vi "DetectCollisionSmoother.vi"(0 "Goal":dbl[](array[numeric]), 4 "Initial State":dbl[](array[numeric]), 6 "enemy_robots":T1[](array[typedef]), 7 "Robot in":T1={"id"=0, "function"=enum."Attacker", "x"=0.0, "y"=0.0, "orientation"=0.0, "v_tangent"=0.0, "v_normal"=0.0, "v_ang"=0.0, "kick_x"=0.0, "kick_z"=0.0, "dribble"=FALSE, "Timestamp"=timestamp(0 s since 1904-01-01), "estimatives"={"est_v_tangent"=0.0, "est_v_normal"=0.0, "est_vx"=0.0, "est_vy"=0.0, "Pos Robot Est"=[]}, "dest_x_kick"=0.0, "dest_y_kick"=0.0, "Gap Coord"=[], "States"=enum."Pass", "Path "=[], "Path  Smooth"=[], "Dest"=[], "vx_desired"=0.0, "vy_desired"=0.0, "slowBehavior"=FALSE, "VSSStates"=enum."Pass"}, 8 "SegmentPointB":dbl[](array[numeric]), 9 "SegmentPointA":dbl[](array[numeric]), 10 "ball":dbl[](array[numeric]), 11 "ignoreBall?":bool) -> (3 "Is there colision?":bool)   [LabVIEW 2023]
uses:
  Vision_class/Old vision/Controls/AI Robot.ctl
  Vision_class/Old vision/Controls/Functions Enum.ctl
  Vision_class/Old vision/Controls/AttackerStates.ctl
  Vision_class/Old vision/Controls/PathDests.ctl
  Vision_class/Old vision/Controls/PathDest.ctl
  Navigation/VSSNavigation/VSSAttackerStates.ctl
panel:
  in  "our_robots":T1[](array[typedef])
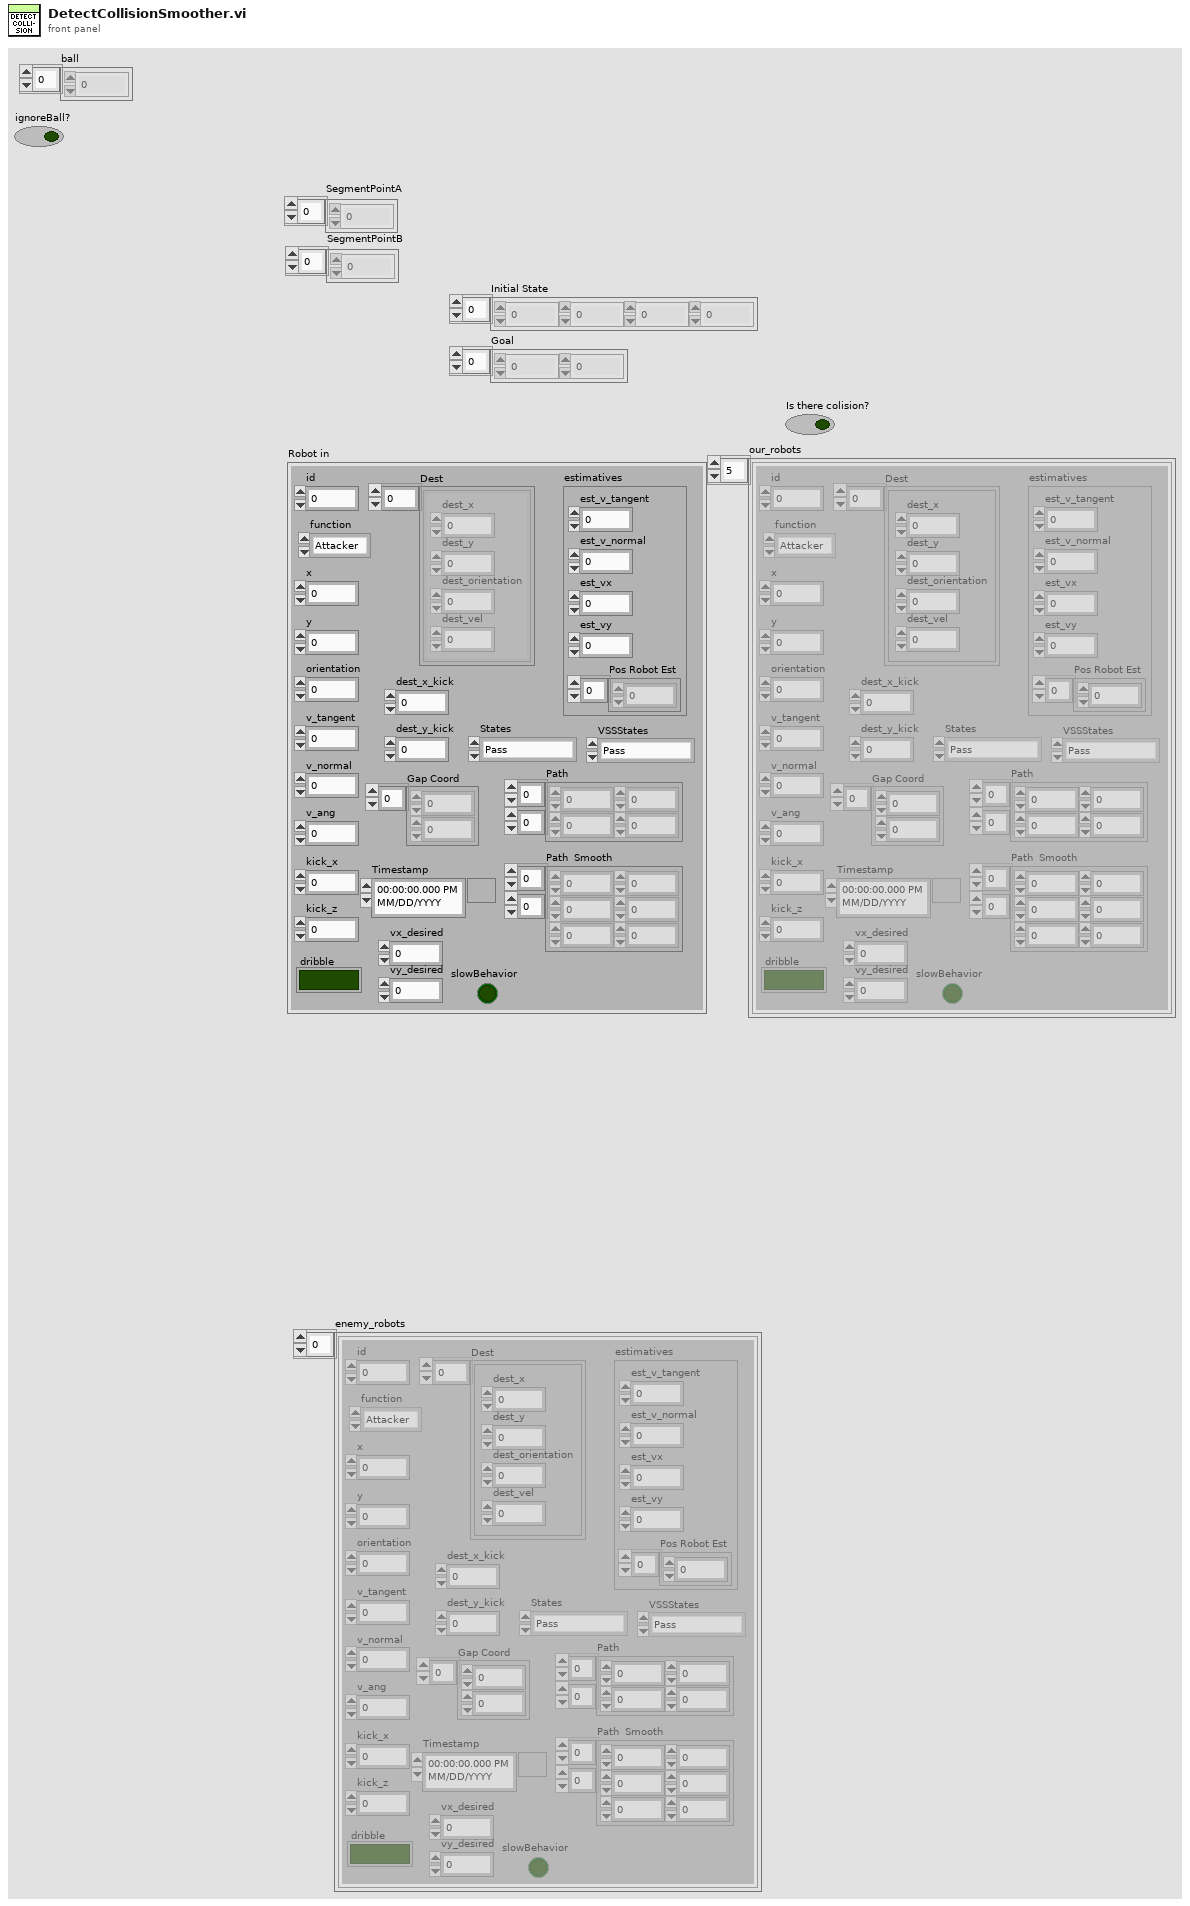
[diagram p1: front panel]
types:
  T1 = typedef "AI Robot.ctl" = cluster{"id":u32, "function":T2, "x":dbl, "y":dbl, "orientation":dbl, "v_tangent":dbl, "v_normal":dbl, "v_ang":dbl, "kick_x":dbl, "kick_z":dbl, "dribble":bool, "Timestamp":timestamp, "estimatives":cluster{"est_v_tangent":dbl, "est_v_normal":dbl, "est_vx":dbl, "est_vy":dbl, "Pos Robot Est":dbl[]}, "dest_x_kick":dbl, "dest_y_kick":dbl, "Gap Coord":dbl[], "States":T3, "Path ":dbl[][], "Path  Smooth":dbl[][], "Dest":T4, "vx_desired":dbl, "vy_desired":dbl, "slowBehavior":bool, "VSSStates":T6}
  T2 = typedef "Functions Enum.ctl" = enum16{"2nd Striker", "Attacker", "Goalie", "Defender", "Striker", "Goto 0", "Dummy", "Kicker", "ZigZag 0", "ZigZag 1", "ZigZag 2", "ZigZag 3", "ZigZag 4", "ZigZag 5", "ZigZag 6", "ZigZag 7", "ZigZag 8", ""}
  T3 = typedef "AttackerStates.ctl" = enum16{"Pass", "GoToTangent", "BallGetting", "GoToKick", ""}
  T4 = typedef "PathDests.ctl" = T5[]
  T5 = typedef "PathDest.ctl" = cluster{"dest_x":dbl, "dest_y":dbl, "dest_orientation":dbl, "dest_vel":dbl}
  T6 = typedef "VSSAttackerStates.ctl" = enum16{"Pass", "GoToTangent", "BallGetting", "GoToKick", "Rotate anti-clockwise", "Rotate Clockwise", ""}
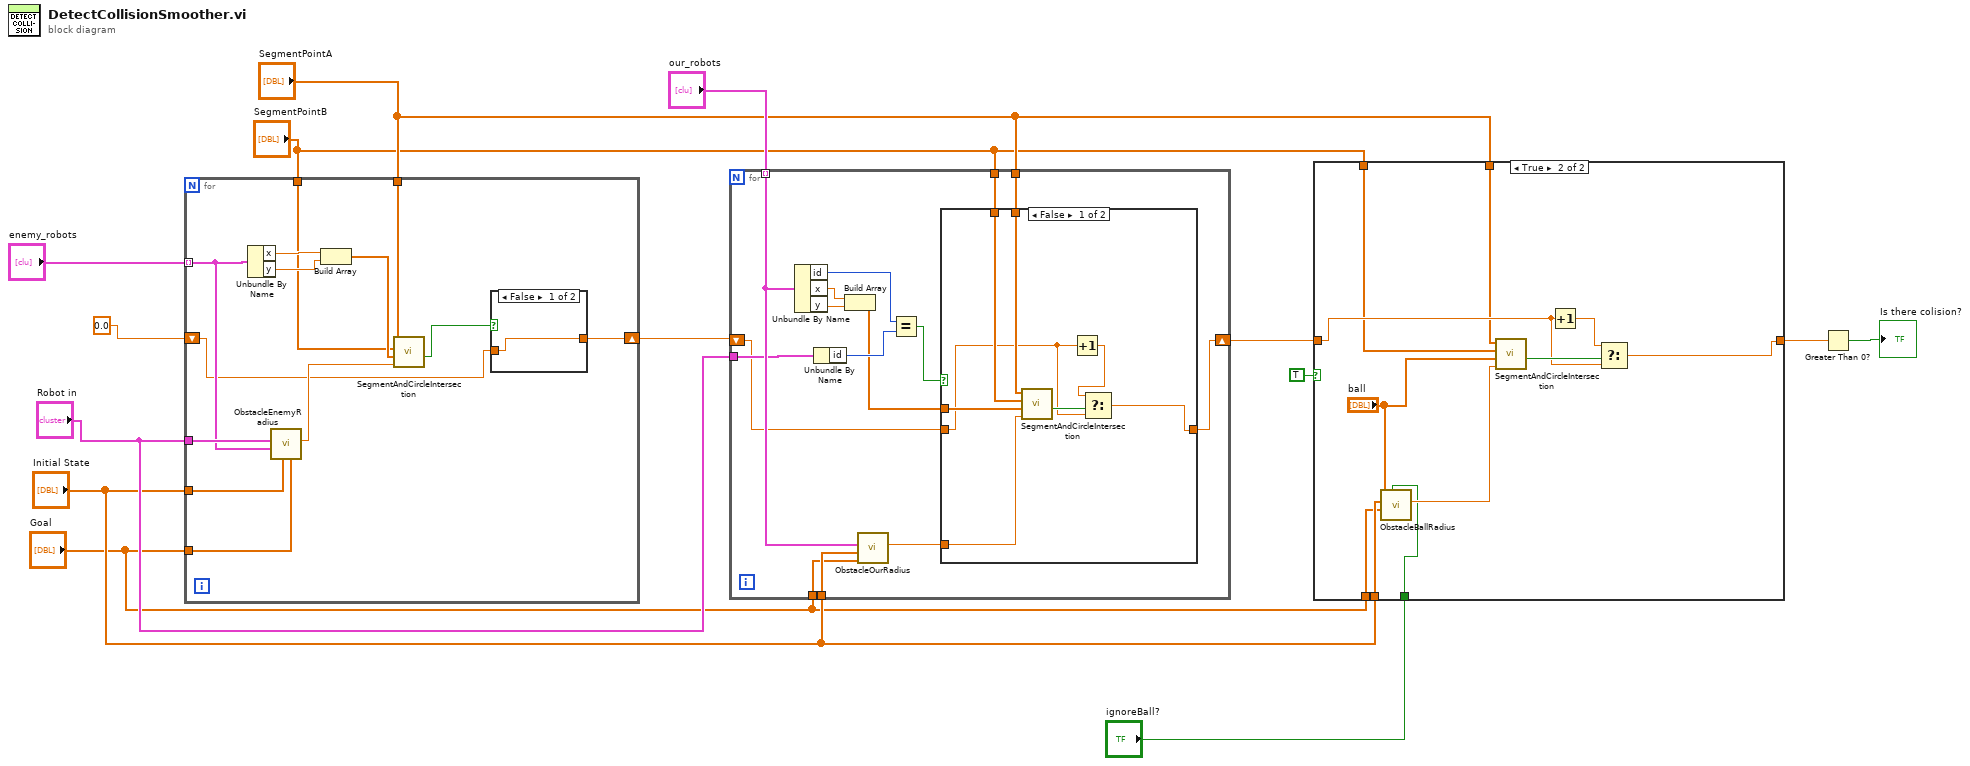
[diagram p0: block diagram]
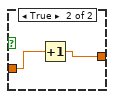
[diagram p4: hidden frame]
diagram:
  n1 = for {
    tunnel: "enemy_robots" -> [w21] mode=indexing
    tunnel: "Initial State" -> [w24]
    tunnel: "Goal" -> [w23]
    tunnel: "Robot in" -> [w22]
    tunnel: "SegmentPointA" -> [w19]
    tunnel: "SegmentPointB" -> [w18]
    shift-right: [w15] -> w10
    shift-left: 0.0 -> [w16]
    n2 = Unbundle By Name(w21) -> ("x"=w27:dbl, "y"=w26:dbl)
    n3 = call "ObstacleEnemyRadius.vi"("Goal"=w23, "Initial State"=w24, "Robot enemy"=w21, "Robot in"=w22) -> ("obstacle enemy radius"=w20:dbl)  [unwired: 7 in]
    n4 = Build Array(w27, w26) -> (w25:dbl[])
    n5 = call "SegmentAndCircleIntersection.vi"("CircleRadius"=w20, "CircleCenter"=w25, "SegmentPointB"=w18, "SegmentPointA"=w19) -> ("DoTheyIntersect?"=w17:bool)  [unwired: 7 in]
    n6 = case shown="False" w17 {
      tunnel: w16 -> [w28 w30]
      tunnel: [w28 w29] -> w15
      frame False {
      }
      frame True {
        n7 = Increment(x=w30) -> (x+1=w29:dbl)
      }
    }
  }
  n8 = for {
    tunnel: "our_robots" -> [w45] mode=indexing
    shift-right: [w38] -> w6
    shift-left: w10 -> [w37]
    tunnel: "Initial State" -> [w44]
    tunnel: "Goal" -> [w43]
    tunnel: "Robot in" -> [w42]
    tunnel: "SegmentPointA" -> [w35]
    tunnel: "SegmentPointB" -> [w34]
    n9 = Unbundle By Name(w45) -> ("id"=w41:u32, "x"=w33:dbl, "y"=w32:dbl)
    n10 = Unbundle By Name(w42) -> ("id"=w40:u32)
    n11 = Build Array(w33, w32) -> (w31:dbl[])
    n12 = call "ObstacleOurRadius.vi"("Goal"=w43, "Initial State"=w44, "other robot"=w45) -> ("obstacle enemy radius"=w36:dbl)  [unwired: 8 in]
    n13 = Equal?(x=w41, y=w40) -> (x = y?=w39:bool)
    n14 = case shown="False" w39 {
      tunnel: [w47 w54] -> w38
      tunnel: w37 -> [w46 w54]
      tunnel: w36 -> [w53 _]
      tunnel: w35 -> [w52 _]
      tunnel: w34 -> [w51 _]
      tunnel: w31 -> [w50 _]
      frame False {
        n15 = call "SegmentAndCircleIntersection.vi"("CircleRadius"=w53, "CircleCenter"=w50, "SegmentPointB"=w51, "SegmentPointA"=w52) -> ("DoTheyIntersect?"=w49:bool)  [unwired: 7 in]
        n16 = Increment(x=w46) -> (x+1=w48:dbl)
        n17 = Select(t=w48, s=w49, f=w46) -> (s? t:f=w47:dbl)
      }
      frame True {
      }
    }
  }
  n18 = case shown="True" TRUE {
    tunnel: [w55 w60] -> w7
    tunnel: w6 -> [w55 w61]
    tunnel: "Initial State" -> [_ w66]
    tunnel: "Goal" -> [_ w65]
    tunnel: "SegmentPointA" -> [_ w59]
    tunnel: "SegmentPointB" -> [_ w58]
    tunnel: "ignoreBall?" -> [_ w56]
    frame False {
    }
    frame True {
      n19 = call "ObstacleBallRadius.vi"("ignoreBall?"=w56, "Goal"=w65, "Initial State"=w66, "ball"="ball") -> ("obstacle enemy radius"=w64:dbl)  [unwired: 7 in]
      n20 = call "SegmentAndCircleIntersection.vi"("CircleRadius"=w64, "CircleCenter"="ball", "SegmentPointB"=w58, "SegmentPointA"=w59) -> ("DoTheyIntersect?"=w63:bool)  [unwired: 7 in]
      n21 = Increment(x=w61) -> (x+1=w62:dbl)
      n22 = Select(t=w62, s=w63, f=w61) -> (s? t:f=w60:dbl)
    }
  }
  n23 = Greater Than 0?(x=w7) -> (x > 0?=→"Is there colision?":bool)
